vi "Configure.vi"(0 "object in":refnum<class "MTEC_Async.lvclass">, 2 "Config Data":T4={"meTEC_CH1_Input Selection (ID 2000)"=2, "meTEC_CH2_Input Selection (ID 2000)"=2, "meTEC_CH1_Object Target Temp. Source Selection (ID 50011)"=0, "meTEC_CH2_Object Target Temp. Source Selection (ID 50011)"=0, "meTEC_CH1_Live Enable (ID 50000)"=0, "meTEC_CH2_Live Enable (ID 50000)"=0, "meTEC_CH1_Object Target Temperature (ID 3000 / 50012) [°C]"=23.0, "meTEC_CH2_Object Target Temperature (ID 3000 / 50012) [°C]"=23.0, "meTEC_CH1_Live Set Current (ID 50001) [A]"=0.0, "meTEC_CH2_Live Set Current (ID 50001) [A]"=0.0, "meTEC_CH1_Live Set Voltage (ID 50002) [V]"=0.0, "meTEC_CH2_Live Set Voltage (ID 50002) [V]"=0.0} {"meTEC_CH2_Live Set Voltage (ID 50002) [V]" min=0.0 max=22.000001907348633 step=0.001 format="%#.3f"; "meTEC_CH1_Live Set Voltage (ID 50002) [V]" min=0.0 max=0.0 step=0.001 format="%#.3f"; "meTEC_CH2_Live Set Current (ID 50001) [A]" min=-10.0 max=10.0 step=0.001 format="%#.3f"; "meTEC_CH1_Live Set Current (ID 50001) [A]" min=0.0 max=0.0 step=0.001 format="%#.3f"; "meTEC_CH2_Object Target Temperature (ID 3000 / 50012) [°C]" min=-273.0 max=1000.0 step=0.001 format="%#.3f"; "meTEC_CH1_Object Target Temperature (ID 3000 / 50012) [°C]" min=0.0 max=0.0 step=0.001 format="%#.3f"; "meTEC_CH2_Live Enable (ID 50000)" items=["Disabled (Reset State)", "Enabled"]; "meTEC_CH1_Live Enable (ID 50000)" items=["Disabled (Reset State)", "Enabled"]; "meTEC_CH2_Object Target Temp. Source Selection (ID 50011)" items=["Parameter ID 3000 (Reset State)", "Parameter ID 50012"]; "meTEC_CH1_Object Target Temp. Source Selection (ID 50011)" items=["Parameter ID 3000 (Reset State)", "Parameter ID 50012"]; "meTEC_CH2_Input Selection (ID 2000)" items=["Static Current / Voltage", "Live Current / Voltage", "Temperature Controller"]; "meTEC_CH1_Input Selection (ID 2000)" items=["Static Current / Voltage", "Live Current / Voltage", "Temperature Controller"]}, 5 "error in (no error)":errorcluster) -> (14 "object out":refnum<class "MTEC_Async.lvclass">, 19 "error out":errorcluster)   [LabVIEW 2019, in "MTEC_Async.lvclass"]
uses:
  MTEC_Async.lvclass
  TEC LabVIEW Control Software v0.14/Source/LV Source/[meerstetter engineering TE Cooling]/TypeDefs/meTEC_ID 2000_Input Selection.ctl
  TEC LabVIEW Control Software v0.14/Source/LV Source/[meerstetter engineering TE Cooling]/TypeDefs/meTEC_ID 50011_Object Target Temperature Source Selection.ctl
  TEC LabVIEW Control Software v0.14/Source/LV Source/[meerstetter engineering TE Cooling]/TypeDefs/meTEC_ID 50000_Live Enable.ctl
  MTEC_Async.lvclass/MTEC_Async.ctl
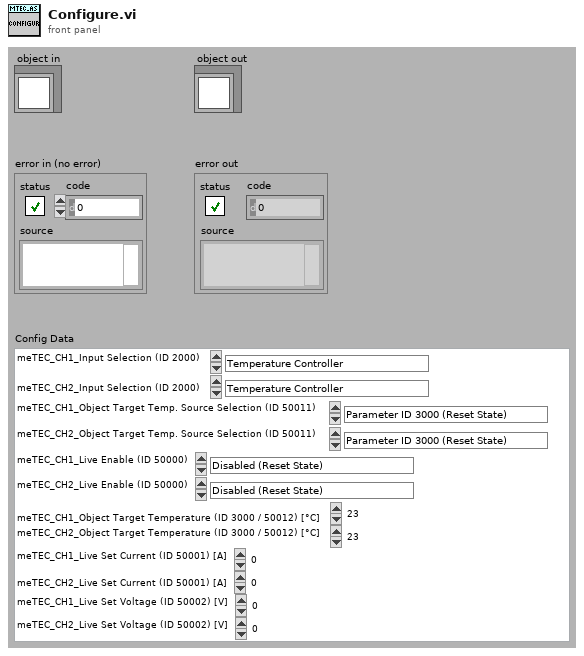
[diagram p1: front panel]
types:
  T1 = typedef "meTEC_ID 2000_Input Selection.ctl" = i32
  T2 = typedef "meTEC_ID 50011_Object Target Temperature Source Selection.ctl" = i32
  T3 = typedef "meTEC_ID 50000_Live Enable.ctl" = i32
  T4 = cluster{"meTEC_CH1_Input Selection (ID 2000)":T1, "meTEC_CH2_Input Selection (ID 2000)":T1, "meTEC_CH1_Object Target Temp. Source Selection (ID 50011)":T2, "meTEC_CH2_Object Target Temp. Source Selection (ID 50011)":T2, "meTEC_CH1_Live Enable (ID 50000)":T3, "meTEC_CH2_Live Enable (ID 50000)":T3, "meTEC_CH1_Object Target Temperature (ID 3000 / 50012) [°C]":dbl, "meTEC_CH2_Object Target Temperature (ID 3000 / 50012) [°C]":dbl, "meTEC_CH1_Live Set Current (ID 50001) [A]":dbl, "meTEC_CH2_Live Set Current (ID 50001) [A]":dbl, "meTEC_CH1_Live Set Voltage (ID 50002) [V]":dbl, "meTEC_CH2_Live Set Voltage (ID 50002) [V]":dbl}
  T5 = cluster{"Message":string, "Message Data":variant}
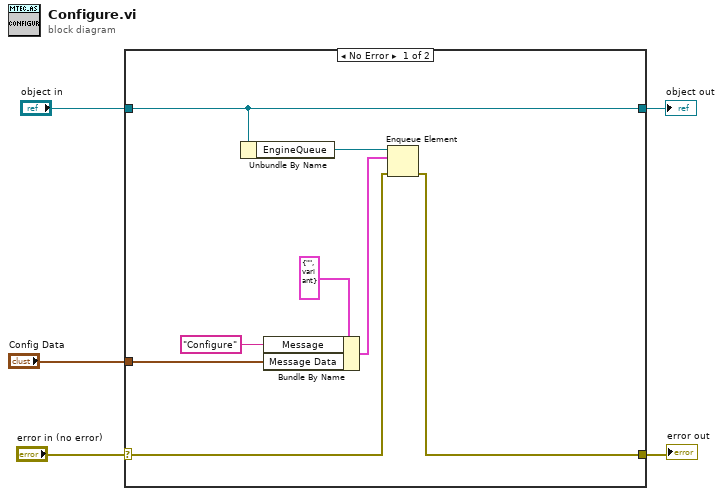
[diagram p0: block diagram]
diagram:
  n1 = case shown="No Error" "error in (no error)" {
    selector: "error in (no error)" -> [w8 w15]
    tunnel: [w7 w15] -> w4
    tunnel: [w13 w14] -> w2
    tunnel: "object in" -> [w13 w14]
    tunnel: "Config Data" -> [w6 _]
    frame No Error {
      n2 = Unbundle By Name(w13) -> ("EngineQueue"=w12:refnum<queue>)
      n3 = Bundle By Name(cluster=T5 {"Message"="", "Message Data"=variant} ("element"), "Message"="Configure", "Message Data"=w6) -> (w9:T5)
      n4 = Enqueue Element(queue=w12, element=w9, error in (no error)=w8) -> (error out=w7:errorcluster)  [unwired: 1 in, 2 out]
    }
    frame Error {
    }
  }
  "error out" <- w4
  "object out" <- w2
